vi "BotSpeak_Tiny.vi"(1 "URAPI":string) -> (2 "URAPI  2":string, 3 "SubsString":string, 4 "Tiny Lines":string[](array[string]))   [LabVIEW 2012]
panel:
  in  "Numeric":u8
  # "1st byte - length\n2nd byte - command\n3rd - nth byte values\n\nvalues are 2 bytes each\n\nNumber - is u16 ( hi byte first)\nOtherwise 8 bit source and 8 bit value\nIf MSB = 1, then it is an array\n\nsources:\n\n200 (C8) - TMR[#]\n201 (C9) - AI[#]\n202 (CA) - DIO[#]\n203 (CB) - PWM[#]\n204 (CC) - SERVO[#]\n\n220 (DC) - TMR[var]\n221 (DD) - AI[var]\n222 (DE) - DIO[var]\n223 (DF) - PWM[var]\n224 (E0) - SERVO[var]\n\n252 (FC) - \n253 (FD) - var[var]\n254 (FE) - \n255 (FF) - var#"
  # "a.. abort\nd.. dump\n+ (x2B).. add\n-*/\n\ng (x67)..get\nG (x47)..goto\nI.. (x49) if\n   < x3C\ni.. not if\nP..ping\nr (x72)..run\nd..debug\nR..run and wait\ns (x73)..script\nE (x45).. end script\ne ... go to ScriptSize\n= (x3D)..set\nW (x57)..wait (ms)\nw (x77)..wait (µs)"
  # "DIO 1,1 - raises port 1 high\nDIO 1 - retrieves the status of DIO 1\nSERVO 1,1.5 - sets servo 1 to 1.5 msec (-1 turns off)\nABORT - stops\nDUMP - gives state of all DIO lines in 2 numbers\nAI 0 - replies with value of channel 0\nAO 0,2.5 - sets PWM out to 50%\nSET test,1.2 - sets variable test to 1.2\nGET test - gets value of variable test\nPING - returns version number\nTIMER 1,"
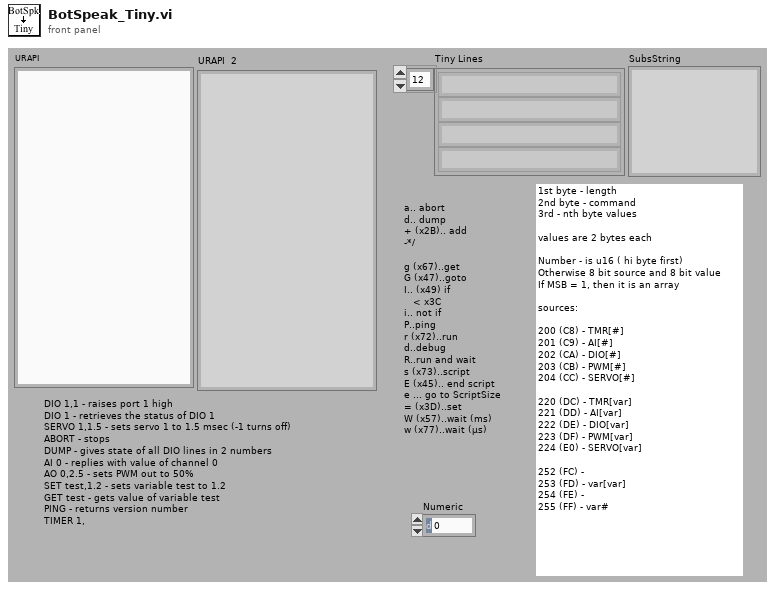
[diagram p1: front panel]
types:
  T1 = cluster{"upper limit":dbl, "lower limit":dbl, "scale":dbl}[]
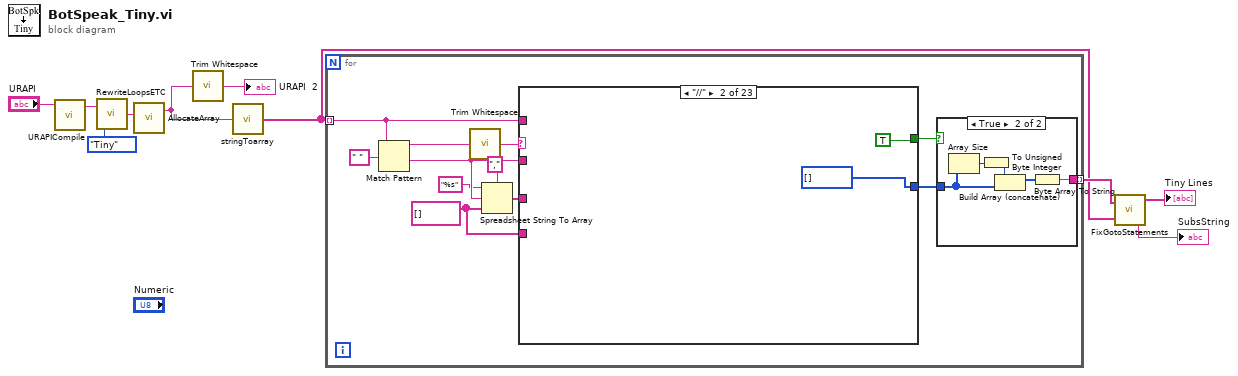
[diagram p0: block diagram]
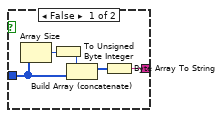
[diagram p2: hidden frame]
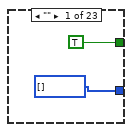
[diagram p3: hidden frame]
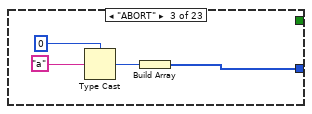
[diagram p4: hidden frame]
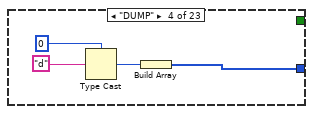
[diagram p5: hidden frame]
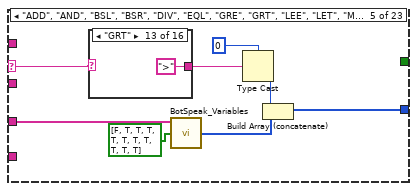
[diagram p6: hidden frame]
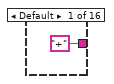
[diagram p7: hidden frame]
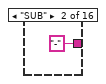
[diagram p8: hidden frame]
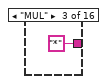
[diagram p9: hidden frame]
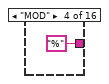
[diagram p10: hidden frame]
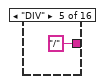
[diagram p11: hidden frame]
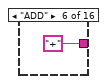
[diagram p12: hidden frame]
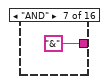
[diagram p13: hidden frame]
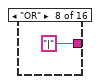
[diagram p14: hidden frame]
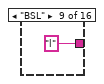
[diagram p15: hidden frame]
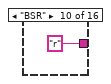
[diagram p16: hidden frame]
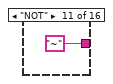
[diagram p17: hidden frame]
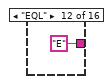
[diagram p18: hidden frame]
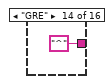
[diagram p19: hidden frame]
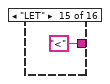
[diagram p20: hidden frame]
diagram:
  n1 = call <userlib>:"URAPICompile.vi"("Script"="URAPI") -> ("trimmed script"=w9:string)  [unwired: 1 in]
  n2 = call <userlib>:"RewriteLoopsETC.vi"("Type"=enum16{"Tiny", "BotSpeak"}."Tiny", "URAPI in"=w9) -> ("URAPI out"=w6:string)
  n3 = call <userlib>:"AllocateArray.vi"("URAPI in"=w6) -> ("URAPI out"=w5:string)  [unwired: 2 in]
  n4 = call <vilib>:"Trim Whitespace.vi"("string"=w5) -> ("trimmed string"=→"URAPI  2":string)  [unwired: 1 in]
  n5 = call <userlib>:"stringToarray.vi"("String"=w5) -> ("Array"=w4:string[])
  n6 = for {
    tunnel: [w15] -> w8 mode=indexing
    tunnel: w4 -> [w11] mode=indexing
    w13 = string[] []
    n7 = Match Pattern(string=w11, regular expression=" ") -> (before substring=w21:string, after substring=w19:string)  [unwired: 1 in, 2 out]
    n8 = call <vilib>:"Trim Whitespace.vi"("string"=w21) -> ("trimmed string"=w20:string)  [unwired: 1 in]
    n9 = Spreadsheet String To Array(delimiter (Tab)=",", format string="%s", spreadsheet string=w19, array type (2D Dbl)=w13) -> (array=w17:string[])
    n10 = case shown="\"//\"" w20 {
      selector: w20 -> [_ _ _ _ w46 _ _ _ _ _ _ _ _ _ _ _ _ _ _ _ _ _ _]
      tunnel: w11 -> [_ _ _ _ _ _ _ _ _ _ _ _ _ _ _ _ _ _ _ _ _ _ w227]
      tunnel: w19 -> [_ _ _ _ _ _ _ _ w108 _ _ _ w145 _ _ _ _ _ _ _ _ _ _]
      tunnel: w17 -> [_ _ _ _ w48 w70 w76 w82 _ _ w124 w130 w139 _ _ w160 w169 w185 w191 w198 w220 w226 _]
      tunnel: [u8[] [] ("unsigned byte array") u8[] [] ("unsigned byte array") w37 w41 w50 w71 w77 w83 w109 w120 w125 w131 w146 w150 w154 w161 w173 w186 w193 w203 w222 w225 w228] -> w16
      tunnel: [TRUE TRUE _ _ _ _ _ _ _ _ _ _ _ _ _ _ _ _ _ _ _ _ _] -> w14
      tunnel: w13 -> [_ _ _ _ _ _ _ _ _ _ _ _ _ _ _ _ _ _ _ _ _ _ _]
      frame "" {
      }
      frame "//" {
      }
      frame "ABORT" {
        n11 = Type Cast(type=u8 0, x="a" ("delimiter (Tab)")) -> (*(type *) &x=w38:u8)
        n12 = Build Array(w38) -> (w37:u8[])
      }
      frame "DUMP" {
        n13 = Type Cast(type=u8 0, x="d" ("delimiter (Tab)")) -> (*(type *) &x=w42:u8)
        n14 = Build Array(w42) -> (w41:u8[])
      }
      frame "ADD", "AND", "BSL", "BSR", "DIV", "EQL", "GRE", "GRT", "LEE", "LET", "MOD", "MUL", "NOT", "OR", "SUB" {
        n15 = case shown="\"GRT\"" w46 {
          tunnel: ["+" ("delimiter (Tab)") "-" ("delimiter (Tab)") "*" ("delimiter (Tab)") "%" ("delimiter (Tab)") "/" ("delimiter (Tab)") "+" ("delimiter (Tab)") "&" ("delimiter (Tab)") "|" ("delimiter (Tab)") "l" ("delimiter (Tab)") "r" ("delimiter (Tab)") "~" ("delimiter (Tab)") "E" ("delimiter (Tab)") ">" ("delimiter (Tab)") "^" ("delimiter (Tab)") "<" ("delimiter (Tab)") "L" ("delimiter (Tab)")] -> w45
          frame Default {
          }
          frame "SUB" {
          }
          frame "MUL" {
          }
          frame "MOD" {
          }
          frame "DIV" {
          }
          frame "ADD" {
          }
          frame "AND" {
          }
          frame "OR" {
          }
          frame "BSL" {
          }
          frame "BSR" {
          }
          frame "NOT" {
          }
          frame "EQL" {
          }
          frame "GRT" {
          }
          frame "GRE" {
          }
          frame "LET" {
          }
          frame "LEE" {
          }
        }
        n16 = call <userlib>:"BotSpeak_Variables.vi"("Var #?"=bool[] [FALSE, TRUE, TRUE, TRUE, TRUE, TRUE, TRUE, TRUE, TRUE, TRUE, TRUE] ("Value of?"), "Variables"=w48) -> ("Binary out"=w51:u8[])  [unwired: 1 in]
        n17 = Type Cast(type=u8 0, x=w45) -> (*(type *) &x=w49:u8)
        n18 = Build Array (concatenate)(w49, w51) -> (w50:u8[])
      }
      frame "GOTO", "goto" {
        n19 = call <userlib>:"BotSpeak_Variables.vi"("Variables"=w70) -> ("Binary out"=w69:u8[])  [unwired: 2 in]
        n20 = Type Cast(type=u8 0, x="G" ("delimiter (Tab)")) -> (*(type *) &x=w72:u8)
        n21 = Build Array (concatenate)(w72, w69) -> (w71:u8[])
      }
      frame "DEBUG" {
        n22 = call <userlib>:"BotSpeak_Variables.vi"("Variables"=w76) -> ("Binary out"=w75:u8[])  [unwired: 2 in]
        n23 = Type Cast(type=u8 0, x="d" ("delimiter (Tab)")) -> (*(type *) &x=w78:u8)
        n24 = Build Array (concatenate)(w78, w75) -> (w77:u8[])
      }
      frame "GOSUB" {
        n25 = call <userlib>:"BotSpeak_Variables.vi"("Variables"=w82) -> ("Binary out"=w81:u8[])  [unwired: 2 in]
        n26 = Type Cast(type=u8 0, x="S" ("delimiter (Tab)")) -> (*(type *) &x=w84:u8)
        n27 = Build Array (concatenate)(w84, w81) -> (w83:u8[])
      }
      frame "IF" {
        w105 = " " ("regular expression")
        w100 = u8 0
        # "will be replaced"
        n28 = Search/Split String(string=w108, search string/char (-)="(" ("regular expression")) -> (substring before match=w95:string, match + rest of string=w90:string)  [unwired: 1 in, 1 out]
        n29 = Search/Split String(string=w90, offset (0)=1) -> (match + rest of string=w88:string)  [unwired: 1 in, 2 out]
        n30 = call <vilib>:"Trim Whitespace.vi"("string"=w95) -> ("trimmed string"=w94:string)  [unwired: 1 in]
        n31 = Match Pattern(string=w88, regular expression=w105) -> (before substring=w101:string, after substring=w106:string)  [unwired: 1 in, 2 out]
        n32 = Match Pattern(string=w106, regular expression=w105) -> (before substring=w99:string, after substring=w104:string)  [unwired: 1 in, 2 out]
        n33 = call <vilib>:"Trim Whitespace.vi"("string"=w99) -> ("trimmed string"=w98:string)  [unwired: 1 in]
        n34 = case shown="\"~\"" w94 {
          tunnel: ["I" ("delimiter (Tab)") "i" ("delimiter (Tab)")] -> w93
          frame Default {
          }
          frame "~" {
          }
        }
        n35 = case shown="\"=\"" w98 {
          tunnel: ["<" ("delimiter (Tab)") "<" ("delimiter (Tab)") ">" ("delimiter (Tab)") "!" ("delimiter (Tab)") "=" ("delimiter (Tab)") "G" ("delimiter (Tab)") "L" ("delimiter (Tab)")] -> w97
          frame Default {
          }
          frame "<" {
          }
          frame ">" {
          }
          frame "!=", "<>" {
          }
          frame "=" {
          }
          frame ">=" {
          }
          frame "<=" {
          }
        }
        n36 = Match Pattern(string=w104, regular expression=")") -> (before substring=w102:string)  [unwired: 1 in, 3 out]
        n37 = Build Array(w101, w102, "0" ("regular expression")) -> (w92:string[])
        n38 = Type Cast(type=w100, x=w97) -> (*(type *) &x=w96:u8)
        n39 = Type Cast(type=w100, x=w93) -> (*(type *) &x=w110:u8)
        n40 = call <userlib>:"BotSpeak_Variables.vi"("Variables"=w92) -> ("Binary out"=w91:u8[])  [unwired: 2 in]
        n41 = Build Array (concatenate)(w110, w96, w91) -> (w109:u8[])
      }
      frame "PING" {
        n42 = Type Cast(type=u8 0, x="P" ("delimiter (Tab)")) -> (*(type *) &x=w121:u8)
        n43 = Build Array(w121) -> (w120:u8[])
      }
      frame "RUN" {
        n44 = call <userlib>:"BotSpeak_Variables.vi"("Variables"=w124) -> ("Binary out"=w126:u8[])  [unwired: 2 in]
        n45 = Type Cast(type=u8 0, x="r" ("delimiter (Tab)")) -> (*(type *) &x=w127:u8)
        n46 = Build Array (concatenate)(w127, w126) -> (w125:u8[])
      }
      frame "RUN&WAIT" {
        n47 = call <userlib>:"BotSpeak_Variables.vi"("Variables"=w130) -> ("Binary out"=w132:u8[])  [unwired: 2 in]
        n48 = Type Cast(type=u8 0, x="R" ("delimiter (Tab)")) -> (*(type *) &x=w133:u8)
        n49 = Build Array (concatenate)(w133, w132) -> (w131:u8[])
      }
      frame "SCRIPT" {
        n50 = Match Pattern(string=w145, regular expression="," ("delimiter (Tab)")) -> (after substring=w141:string)  [unwired: 1 in, 3 out]
        n51 = Match Pattern(string=w141, regular expression="," ("delimiter (Tab)")) -> (after substring=w140:string)  [unwired: 1 in, 3 out]
        n52 = Array Subset(array=w139, length=2) -> (w137:string[])  [unwired: 1 in]
        n53 = call <userlib>:"BotSpeak_Variables.vi"("Variables"=w137) -> ("Binary out"=w136:u8[])  [unwired: 2 in]
        n54 = String To Byte Array(string=w140) -> (unsigned byte array=w143:u8[])
        n55 = Type Cast(type=u8 0, x="s" ("delimiter (Tab)")) -> (*(type *) &x=w147:u8)
        n56 = Build Array (concatenate)(w147, w136, w143) -> (w146:u8[])
      }
      frame "ENDSCRIPT" {
        n57 = Type Cast(type=u8 0, x="E" ("delimiter (Tab)")) -> (*(type *) &x=w151:u8)
        n58 = Build Array(w151) -> (w150:u8[])
      }
      frame "END", "end" {
        n59 = Type Cast(type=u8 0, x="e" ("delimiter (Tab)")) -> (*(type *) &x=w155:u8)
        n60 = Build Array(w155) -> (w154:u8[])
      }
      frame "SERVO" {
        n61 = Type Cast(type=u8 0, x="S" ("delimiter (Tab)")) -> (*(type *) &x=w162:u8)
        n62 = call <userlib>:"BotSpeak_Variables.vi"("Scaling"=T1 [{"upper limit"=0.0, "lower limit"=0.0, "scale"=0.0}, {"upper limit"=3.0, "lower limit"=0.0, "scale"=180.0}], "Variables"=w160) -> ("Binary out"=w158:u8[])  [unwired: 1 in]
        n63 = Build Array (concatenate)(w162, w158) -> (w161:u8[])
      }
      frame "SET" {
        n64 = Index Array(array=w169) -> (element=w168:string)  [unwired: 1 in]
        n65 = Match Pattern(string=w168, regular expression="\\[") -> (before substring=w166:string)  [unwired: 1 in, 3 out]
        n66 = case shown="Default" w166 {
          tunnel: [T1 [{"upper limit"=0.0, "lower limit"=0.0, "scale"=1.0}, {"upper limit"=0.0, "lower limit"=0.0, "scale"=1.0}, {"upper limit"=0.0, "lower limit"=0.0, "scale"=1.0}, {"upper limit"=0.0, "lower limit"=0.0, "scale"=1.0}, {"upper limit"=0.0, "lower limit"=0.0, "scale"=1.0}, {"upper limit"=0.0, "lower limit"=0.0, "scale"=1.0}, {"upper limit"=0.0, "lower limit"=0.0, "scale"=1.0}, {"upper limit"=0.0, "lower limit"=0.0, "scale"=1.0}, {"upper limit"=0.0, "lower limit"=0.0, "scale"=1.0}, {"upper limit"=0.0, "lower limit"=0.0, "scale"=1.0}, {"upper limit"=0.0, "lower limit"=0.0, "scale"=1.0}] ("Scaling") T1 [{"upper limit"=1.0, "lower limit"=0.0, "scale"=1.0}, {"upper limit"=100.0, "lower limit"=0.0, "scale"=100.0}, {"upper limit"=1.0, "lower limit"=0.0, "scale"=1.0}, {"upper limit"=0.0, "lower limit"=0.0, "scale"=1.0}, {"upper limit"=0.0, "lower limit"=0.0, "scale"=1.0}, {"upper limit"=0.0, "lower limit"=0.0, "scale"=1.0}, {"upper limit"=0.0, "lower limit"=0.0, "scale"=1.0}, {"upper limit"=0.0, "lower limit"=0.0, "scale"=1.0}, {"upper limit"=0.0, "lower limit"=0.0, "scale"=1.0}, {"upper limit"=0.0, "lower limit"=0.0, "scale"=1.0}, {"upper limit"=0.0, "lower limit"=0.0, "scale"=1.0}] ("Scaling") T1 [{"upper limit"=1.0, "lower limit"=0.0, "scale"=1.0}, {"upper limit"=2.0, "lower limit"=1.0, "scale"=100.0}, {"upper limit"=0.0, "lower limit"=0.0, "scale"=1.0}, {"upper limit"=0.0, "lower limit"=0.0, "scale"=1.0}, {"upper limit"=0.0, "lower limit"=0.0, "scale"=1.0}, {"upper limit"=0.0, "lower limit"=0.0, "scale"=1.0}, {"upper limit"=0.0, "lower limit"=0.0, "scale"=1.0}, {"upper limit"=0.0, "lower limit"=0.0, "scale"=1.0}, {"upper limit"=0.0, "lower limit"=0.0, "scale"=1.0}, {"upper limit"=0.0, "lower limit"=0.0, "scale"=1.0}, {"upper limit"=0.0, "lower limit"=0.0, "scale"=1.0}] ("Scaling") T1 [{"upper limit"=0.0, "lower limit"=0.0, "scale"=1.0}, {"upper limit"=1.0, "lower limit"=0.0, "scale"=1.0}, {"upper limit"=0.0, "lower limit"=0.0, "scale"=1.0}, {"upper limit"=0.0, "lower limit"=0.0, "scale"=1.0}, {"upper limit"=0.0, "lower limit"=0.0, "scale"=1.0}, {"upper limit"=0.0, "lower limit"=0.0, "scale"=1.0}, {"upper limit"=0.0, "lower limit"=0.0, "scale"=1.0}, {"upper limit"=0.0, "lower limit"=0.0, "scale"=1.0}, {"upper limit"=0.0, "lower limit"=0.0, "scale"=1.0}, {"upper limit"=0.0, "lower limit"=0.0, "scale"=1.0}, {"upper limit"=0.0, "lower limit"=0.0, "scale"=1.0}] ("Scaling")] -> w165
          frame Default {
          }
          frame "PWM" {
          }
          frame "SERVO" {
          }
          frame "DIO" {
          }
        }
        n67 = Type Cast(type=u8 0, x="=" ("delimiter (Tab)")) -> (*(type *) &x=w172:u8)
        n68 = call <userlib>:"BotSpeak_Variables.vi"("Scaling"=w165, "Var #?"=bool[] [TRUE, TRUE, TRUE, TRUE, TRUE, TRUE, TRUE, TRUE, TRUE, TRUE, TRUE] ("Value of?"), "Variables"=w169) -> ("Binary out"=w170:u8[])
        n69 = Build Array (concatenate)(w172, w170) -> (w173:u8[])
      }
      frame "SYSTEM" {
        n70 = call <userlib>:"BotSpeak_Variables.vi"("Var #?"=bool[] [TRUE, TRUE, TRUE, TRUE, TRUE, TRUE, TRUE, TRUE, TRUE, TRUE, TRUE] ("Value of?"), "Variables"=w185) -> ("Binary out"=w182:u8[])  [unwired: 1 in]
        n71 = Array Size(array=w182) -> (size(s)=w181:i32)
        n72 = Type Cast(type=u8 0, x="!" ("delimiter (Tab)")) -> (*(type *) &x=w183:u8)
        n73 = To Unsigned Byte Integer(number=w181) -> (unsigned 8bit integer=w180:u8)
        n74 = Build Array (concatenate)(w183, w180, w182) -> (w186:u8[])
      }
      frame "GET" {
        n75 = Type Cast(type=u8 0, x="g" ("delimiter (Tab)")) -> (*(type *) &x=w192:u8)
        n76 = call <userlib>:"BotSpeak_Variables.vi"("Var #?"=bool[] [TRUE, TRUE, TRUE, TRUE, TRUE, TRUE, TRUE, TRUE, TRUE, TRUE, TRUE] ("Value of?"), "Variables"=w191) -> ("Binary out"=w189:u8[])  [unwired: 1 in]
        n77 = Build Array (concatenate)(w192, w189) -> (w193:u8[])
      }
      frame "WAIT" {
        n78 = Index Array(array=w198) -> (element=w201:string)  [unwired: 1 in]
        n79 = Scan From String(input string=w201) -> (error out=w200:errorcluster, output 1=w199:dbl)  [unwired: 4 in, 2 out]
        n80 = case shown="No Error" w200 {
          tunnel: [w207 "W" ("delimiter (Tab)")] -> w202
          tunnel: w199 -> [w211 _]
          tunnel: w198 -> [_ _]
          tunnel: [w206 T1 [{"upper limit"=0.0, "lower limit"=0.0, "scale"=1.0}] ("Scaling")] -> w196
          frame No Error {
            n81 = Absolute Value(x=w211) -> (abs(x)=w210:dbl)
            n82 = Less?(x=w210, y=0.01) -> (x < y?=w208:bool)
            n83 = case shown="True" w208 {
              tunnel: ["w" ("delimiter (Tab)") "W" ("delimiter (Tab)")] -> w207
              tunnel: [T1 [{"upper limit"=0.0, "lower limit"=0.0, "scale"=1000000.0}] ("Scaling") T1 [{"upper limit"=0.0, "lower limit"=0.0, "scale"=1000.0}] ("Scaling")] -> w206
              frame True {
              }
              frame False {
              }
            }
          }
          frame Error {
            # "variable for wait time\n(in msec)"
          }
        }
        n84 = Type Cast(type=u8 0, x=w202) -> (*(type *) &x=w204:u8)
        n85 = call <userlib>:"BotSpeak_Variables.vi"("Scaling"=w196, "Variables"=w198) -> ("Binary out"=w197:u8[])  [unwired: 1 in]
        n86 = Build Array (concatenate)(w204, w197) -> (w203:u8[])
      }
      frame "WAITµs" {
        n87 = call <userlib>:"BotSpeak_Variables.vi"("Scaling"=T1 [{"upper limit"=0.0, "lower limit"=0.0, "scale"=1.0}], "Variables"=w220) -> ("Binary out"=w218:u8[])  [unwired: 1 in]
        n88 = Type Cast(type=u8 0, x="w" ("delimiter (Tab)")) -> (*(type *) &x=w223:u8)
        n89 = Build Array (concatenate)(w223, w218) -> (w222:u8[])
      }
      frame "convert" {
        n90 = call <userlib>:"BotSpeak_Variables.vi"("Variables"=w226) -> ("Binary out"=w225:u8[])  [unwired: 2 in]
      }
      frame Default {
        n91 = String To Byte Array(string=w227) -> (unsigned byte array=w228:u8[])
      }
    }
    n92 = case shown="True" w14 {
      tunnel: w16 -> [w25 w30]
      tunnel: [w27 w32] -> w15
      frame False {
        n93 = Array Size(array=w25) -> (size(s)=w26:i32)
        n94 = To Unsigned Byte Integer(number=w26) -> (unsigned 8bit integer=w23:u8)
        n95 = Build Array (concatenate)(w23, w25) -> (w24:u8[])
        n96 = Byte Array To String(unsigned byte array=w24) -> (string=w27:string)
      }
      frame True {
        n97 = Array Size(array=w30) -> (size(s)=w31:i32)
        n98 = To Unsigned Byte Integer(number=w31) -> (unsigned 8bit integer=w28:u8)
        n99 = Build Array (concatenate)(w28, w30) -> (w29:u8[])
        n100 = Byte Array To String(unsigned byte array=w29) -> (string=w32:string)
      }
    }
  }
  n101 = call <userlib>:"FixGotoStatements.vi"("URAPI LInes"=w4, "Tiny Lines"=w8) -> ("SubsString"=→"SubsString":string, "Tiny Fixed"=→"Tiny Lines":string[])  [unwired: 1 out]
